vi "Get SMO Database Paths.vi"(5 "getAll Cluster":variant, 7 "Default Paths":string, 8 "error in (no error)":errorcluster, 11 "Instrument in":refnum<class "Instrument.lvclass">) -> (0 "error out":errorcluster, 2 "Paths":string, 3 "Instrument out":refnum<class "Instrument.lvclass">)   [LabVIEW 2019, in "Instrument.lvlib" / "Instrument.lvclass"]
doc: "Override this VI to return a list of paths for logging data"
uses:
  Instrument.lvclass
  Instrument.lvclass/Instrument.ctl
  <userlib>/LevyLab/LV-Data/LV-Data.PG/LV-Data.PGSQL.lvclass
  <vilib>/Utility/Data Type/NI_Data Type.lvlib
  <userlib>/LevyLab/LV-Data/LV-Data.PG/API/Write Variable (one-row).vi
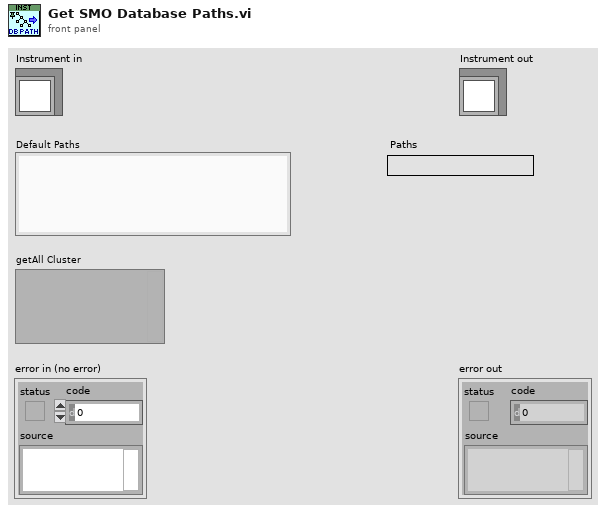
[diagram p1: front panel]
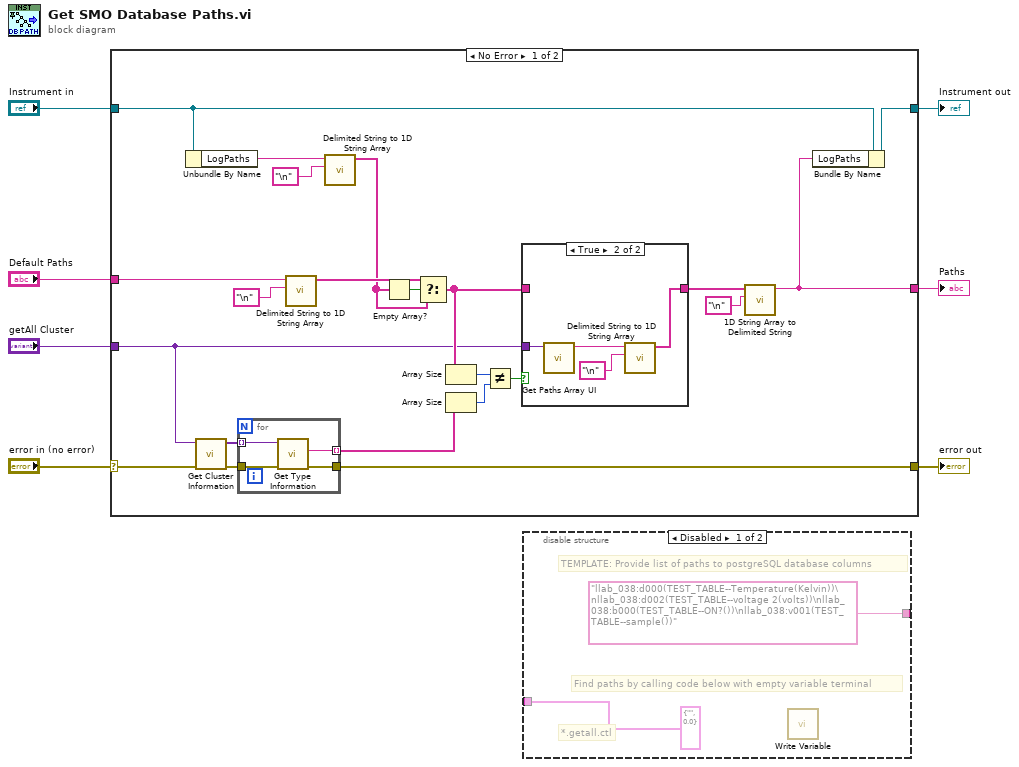
[diagram p0: block diagram]
diagram:
  n1 = case shown="No Error" "error in (no error)" {
    selector: "error in (no error)" -> [w17 w40]
    tunnel: [w20 w40] -> w6
    tunnel: [w28 w39] -> w4
    tunnel: "Instrument in" -> [w29 w39]
    tunnel: "Default Paths" -> [w12 _]
    tunnel: [w14 _] -> w2
    tunnel: "getAll Cluster" -> [w19 _]
    frame No Error {
      n2 = Unbundle By Name(w29) -> ("LogPaths"=w9:string)
      n3 = call <vilib>:"Get Cluster Information.vi"("error in (no error)"=w17, "variant"=w19) -> ("error out"=w21:errorcluster, "cluster elements"=w22:variant[])  [unwired: 8 in]
      n4 = for {
        tunnel: w22 -> [w33] mode=indexing
        tunnel: w21 -> [w32]
        tunnel: [w31] -> w20
        tunnel: [w30] -> w18 mode=indexing
        n5 = call <vilib>:"Get Type Information.vi"("error in (no error)"=w32, "variant"=w33) -> ("error out"=w31:errorcluster, "name"=w30:string)  [unwired: 5 in, 3 out]
      }
      n6 = call <vilib>:"Delimited String to 1D String Array.vi"("delimiter"="\n" ("delimiter (Tab)"), "delimited string"=w12) -> ("string array"=w11:string[])  [unwired: 9 in]
      n7 = call <vilib>:"Delimited String to 1D String Array.vi"("delimiter"="\n" ("delimiter (Tab)"), "delimited string"=w9) -> ("string array"=w8:string[])  [unwired: 9 in]
      n8 = Empty Array?(array=w8) -> (empty?=w27:bool)
      n9 = Select(t=w11, s=w27, f=w8) -> (s? t:f=w24:string[])
      n10 = Array Size(array=w24) -> (size(s)=w23:i32)
      n11 = Array Size(array=w18) -> (size(s)=w26:i32)
      n12 = Not Equal?(x=w23, y=w26) -> (x != y?=w25:bool)
      n13 = case shown="True" w25 {
        tunnel: w19 -> [_ w38]
        tunnel: [w34 w35] -> w16
        tunnel: w24 -> [w34 _]
        frame False {
        }
        frame True {
          n14 = call <userlib>:"Get Paths Array UI.vi"("Data"=w38) -> ("selected_paths"=w36:string)  [unwired: 9 in, 1 out]
          n15 = call <vilib>:"Delimited String to 1D String Array.vi"("delimiter"="\n" ("delimiter (Tab)"), "delimited string"=w36) -> ("string array"=w35:string[])  [unwired: 9 in]
        }
      }
      n16 = call <vilib>:"1D String Array to Delimited String.vi"("delimiter"="\n" ("delimiter (Tab)"), "string array"=w16) -> ("delimited string"=w14:string)  [unwired: 9 in]
      n17 = Bundle By Name(cluster=w29, "LogPaths"=w14) -> (w28:refnum<class "Instrument.lvclass">)
    }
    frame Error {
    }
  }
  "error out" <- w6
  "Instrument out" <- w4
  "Paths" <- w2
  n18 = disable-structure shown="Disabled" {
    disable-tunnel: ["llab_038:d000(TEST_TABLE--Temperature(Kelvin))\nllab_038:d002(TEST_TABLE--voltage 2(volts))\nllab_038:b000(TEST_TABLE--ON?())\nllab_038:v001(TEST_TABLE--sample())" ("Paths") _] -> _
    disable-tunnel: [cluster{string, dbl} {"", 0.0} _] -> _
    frame Disabled {
      # "Find paths by calling code below with empty variable terminal"
      # "*.getall.ctl"
      # "TEMPLATE: Provide list of paths to postgreSQL database columns"
      n19 = call-poly <userlib>:"Write Variable.vi"() -> ()  [unwired: 8 in, 4 out]
    }
    frame Enabled {
    }
  }
